vi "AES APU Degrees per Tick.vi"(9 "Top-Level Clock Rate (40 MHz)":dbl=40000000.0, 11 "RPM":dbl format="%#_15g") -> (2 "degrees per tick":fxp<+/-,47,-4> format="%.50g", 3 "Actual RPM":dbl format="%#_20g")   [LabVIEW 2010, in "AES.lvlib" / "AES RT.lvlib"]
doc: "This VI takes the RPM as an input and calculates the degrees of rotation the crank moves per tick of the FPGA clock. The degrees per tick calculated is then passed to the FPGA to be used by the Crank Angle and Output.vi in order to generate the crank output at the correct RPM. The Actual RPM which is derived from the degrees per tick is also returned. The Actual RPM may be slightly different than the RPM requested because of the precision of degrees per tick and the FPGA's Top-Level Clock Rate."
uses:
  AES RT.lvlib
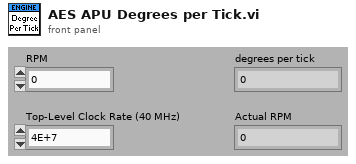
[diagram p1: front panel]
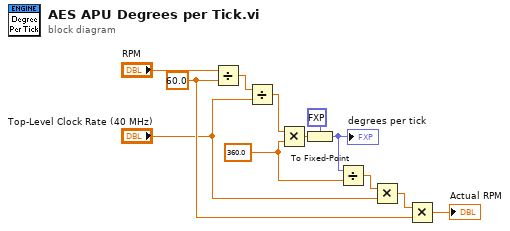
[diagram p0: block diagram]
diagram:
  w12 = 360.0 ("y")
  w8 = 60.0 ("y")
  n1 = Divide(x="RPM", y=w8) -> (x/y=w2:dbl)
  n2 = Divide(x=w2, y="Top-Level Clock Rate (40 MHz)") -> (x/y=w3:dbl)
  n3 = Multiply(x=w3, y=w12) -> (x*y=w5:dbl)
  n4 = To Fixed-Point(fixed-point type=fxp<+/-,47,-4> 0.0 ("Degrees/Tooth"), number=w5) -> (fixed-point=w10:fxp<+/-,47,-4>)
  "degrees per tick" <- w10
  n5 = Divide(x=w10, y=w12) -> (x/y=w11:dbl)
  n6 = Multiply(x=w11, y="Top-Level Clock Rate (40 MHz)") -> (x*y=w7:dbl)
  n7 = Multiply(x=w7, y=w8) -> (x*y=→"Actual RPM":dbl)
